vi "cdaq_anal_close.vi"(8 "error in":errorcluster, 11 "cdaq session in":T1={"mclk [Hz]"=12800000.0, "DAC device"="", "ADC device"="", "DAC task"="", "ADC task"="", "adc idn"="", "dac idn"="", "fs [Hz]"=50000.0, "queue adc cmd"=refnum, "queue adc data"=refnum, "adc proc ref"=refnum}) -> (0 "error out":errorcluster, 3 "cdaq session out":T1={"mclk [Hz]"=12800000.0, "DAC device"="", "ADC device"="", "DAC task"="", "ADC task"="", "adc idn"="", "dac idn"="", "fs [Hz]"=50000.0, "queue adc cmd"=refnum, "queue adc data"=refnum, "adc proc ref"=refnum})   [LabVIEW 2013]
uses:
  cdaq_anal_session.ctl
  cdaq_anal_adc_command.ctl
  cdaq_anal_adc_data.ctl
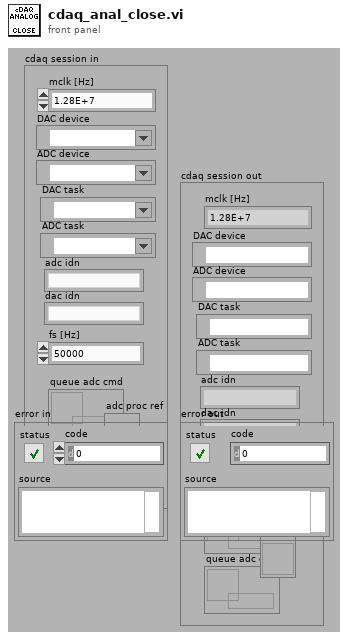
[diagram p1: front panel]
types:
  T1 = typedef "cdaq_anal_session.ctl" = cluster{"mclk [Hz]":dbl, "DAC device":tag, "ADC device":tag, "DAC task":refnum<k21>, "ADC task":refnum<k21>, "adc idn":string, "dac idn":string, "fs [Hz]":dbl, "queue adc cmd":refnum<queue>, "queue adc data":refnum<queue>, "adc proc ref":refnum<vi>}
  T2 = typedef "cdaq_anal_adc_command.ctl" = cluster{"sample to get":i32, "stop":bool}
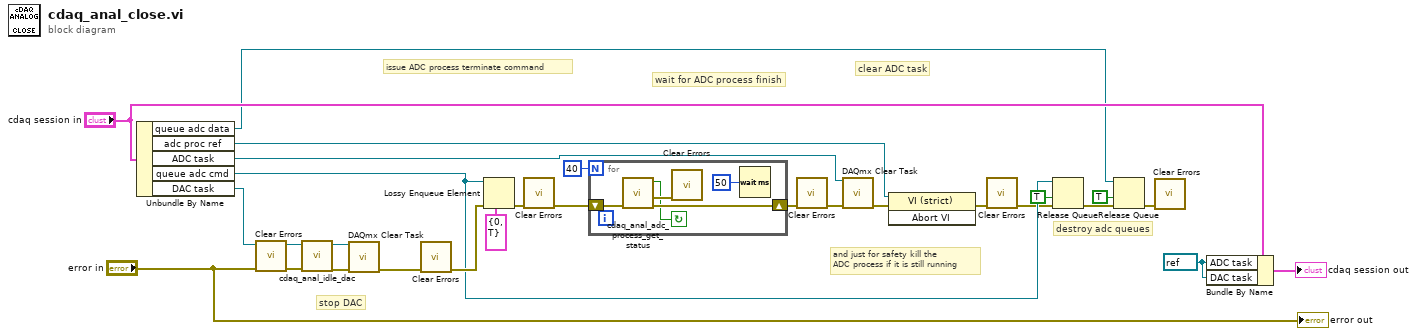
[diagram p0: block diagram]
diagram:
  w26 = refnum<k21> refnum ("ADC task")
  # "destroy adc queues"
  # "and just for safety kill the\nADC process if it is still running"
  # "clear ADC task"
  # "wait for ADC process finish"
  # "issue ADC process terminate command"
  # "stop DAC"
  n1 = Unbundle By Name("cdaq session in") -> ("queue adc data"=w5:refnum<queue>, "adc proc ref"=w11:refnum<vi>, "ADC task"=w15:refnum<k21>, "queue adc cmd"=w8:refnum<queue>, "DAC task"=w24:refnum<k21>)
  n2 = call <vilib>:"Clear Errors.vi"("error in (no error)"="error in") -> ("error out"=w14:errorcluster)  [unwired: 6 in]
  n3 = call "cdaq_anal_idle_dac.vi"("error in"=w14, "task in"=w24) -> ("error out"=w22:errorcluster, "task out"=w23:refnum<k21>)  [unwired: 8 in]
  n4 = call <vilib>:"DAQmx Clear Task.vi"("task in"=w23, "error in"=w22) -> ("error out"=w13:errorcluster)  [unwired: 13 in]
  n5 = call <vilib>:"Clear Errors.vi"("error in (no error)"=w13) -> ("error out"=w12:errorcluster)  [unwired: 6 in]
  n6 = Lossy Enqueue Element(queue=w8, element=T2 {"sample to get"=0, "stop"=TRUE}, error in (no error)=w12) -> (error out=w20:errorcluster)  [unwired: 3 out]
  n7 = call <vilib>:"Clear Errors.vi"("error in (no error)"=w20) -> ("error out"=w19:errorcluster)  [unwired: 6 in]
  n8 = for {
    N: 40 -> [_]
    shift-right: [w31] -> w17
    shift-left: w19 -> [w32]
    stop <- w29 continue-if-true
    n9 = call "cdaq_anal_adc_process_get_status.vi"("error in"=w32) -> ("error out"=w31:errorcluster, "sweep error out"=w30:errorcluster, "is running"=w29:bool)  [unwired: 8 in]
    n10 = call <vilib>:"Clear Errors.vi"("error in (no error)"=w30) -> ()  [unwired: 6 in, 1 out]
    n11 = Wait (ms)(milliseconds to wait=u32 50) -> ()  [unwired: 1 out]
  }
  n12 = call <vilib>:"Clear Errors.vi"("error in (no error)"=w17) -> ("error out"=w16:errorcluster)  [unwired: 6 in]
  n13 = call <vilib>:"DAQmx Clear Task.vi"("task in"=w15, "error in"=w16) -> ("error out"=w10:errorcluster)  [unwired: 13 in]
  n14 = invoke class="VI (strict)" method="Abort VI"(reference=w11, error in=w10) -> (error out=w3:errorcluster)  [unwired: 1 in, 2 out]
  n15 = call <vilib>:"Clear Errors.vi"("error in (no error)"=w3) -> ("error out"=w2:errorcluster)  [unwired: 6 in]
  n16 = Release Queue(queue=w8, force destroy? (F)=TRUE, error in (no error)=w2) -> (error out=w6:errorcluster)  [unwired: 2 out]
  n17 = Release Queue(queue=w5, force destroy? (F)=TRUE, error in (no error)=w6) -> (error out=w1:errorcluster)  [unwired: 2 out]
  n18 = call <vilib>:"Clear Errors.vi"("error in (no error)"=w1) -> ()  [unwired: 6 in, 1 out]
  n19 = Bundle By Name(cluster="cdaq session in", "ADC task"=w26, "DAC task"=w26) -> (→"cdaq session out":T1)
  "error out" <- "error in"
